vi "getMdfType.vi"() -> (3 "mdfType":i32(ring) items=["Mdf3Basic", "Mdf4Basic", "MdfBusLogger", "MdfConverter"])   [LabVIEW 2025, in "MdfFile.lvlib"]
uses:
  MdfFile.lvlib
  data/mdflibrary.dll
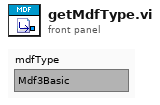
[diagram p1: front panel]
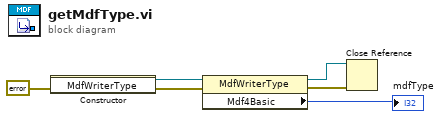
[diagram p0: block diagram]
diagram:
  n1 = constructor class="MdfWriterType"(error in=errorcluster {"status"=FALSE, "code"=0, "source"=""} ("error in (no error)")) -> (reference out=w6:refnum<k24>, error out=w5:errorcluster)  [unwired: 2 in, 1 out]
  n2 = property class="MdfWriterType"(reference=w6, error in=w5) -> (reference out=w4:refnum<k24>, error out=w3:errorcluster, "Mdf4Basic"=→"mdfType":i32)
  n3 = Close Reference(reference=w4, error in (no error)=w3) -> ()  [unwired: 1 out]
